vi "GetPressureAtMouse XYGraph.vi"(2 "Coords":T1, 3 "GraphRefnum":refnum<vi>) -> (0 "Numeric":dbl, 1 "String":string)   [LabVIEW 2013, in "main.lvlib"]
uses:
  main.lvlib
  <vilib>/Utility/miscctls.llb/LVPoint32TypeDef.ctl
  Controls/Enum Globals.ctl
  Controls/Enum Variables.ctl
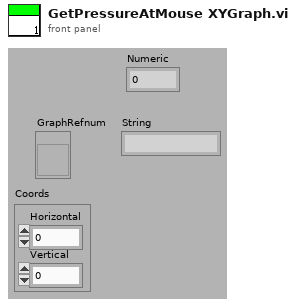
[diagram p1: front panel]
types:
  T1 = typedef "LVPoint32TypeDef.ctl" = cluster{"Horizontal":i32, "Vertical":i32}
  T2 = typedef "main.lvlib/Enum Variables.ctl" = enum16{"SetAcqFilter", "GetAcqFilter", "Set Filter", "Get Filter", "Set Height", "Get Height", "Set Blue Pressure", "Get Blue Pressure", "Set Red Pressure", "Get Red Pressure", "Init", "Reset Pressure", "Set Red Cursors", "Get Red Cursors", "Set Blue Cursors", "Get Blue Cursors", "Set Language", "Get Language", "Set Active Graphs", "Get ActiveGraphs", "Set Method", "Get Method", "Set Encryption", "Get Encryption", "Set ExcelVersion", "Get ExcelVersion", "Set DICOM Avail", "Get DICOM Avail", "Set DICOM Encode", "Get DICOM Encode", "Set JournalExport", "Get JournalExport", "Set Sequence", "Get Sequence", "Set DAQ Connected", "Get DAQ Connected", "Set Current Graph", "Get Current Graph", "Set General Settings", "Get Hyphenation", "Set Arm Calc Method", "Get Arm Calc Method", "Set Dicom Tags", "Get Dicom Tags", "Set BT Serial", "Get BT Serial", "Set BT Accepted Serials", "Get BT Accepted Serials", "Get BT License", "Set BT License"}
  T3 = typedef "main.lvlib/Enum Globals.ctl" = enum16{"Init", "Set DataPath", "Set Freq", "Get"}
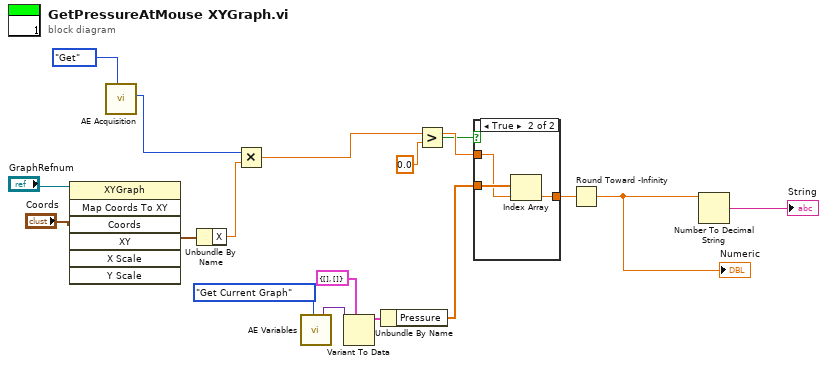
[diagram p0: block diagram]
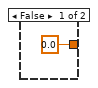
[diagram p2: hidden frame]
diagram:
  n1 = invoke class="XYGraph" method="Map Coords To XY"(reference="GraphRefnum", "Coords"="Coords") -> ("XY"=w14:cluster{"X":dbl, "Y":dbl})  [unwired: 5 in, 6 out]
  n2 = call "AE Acquisition.vi"("Action"=Enum_Globals."Get") -> ("Freq Out"=w7:i32)  [unwired: 7 in, 3 out]
  n3 = Unbundle By Name(w14) -> ("X"=w15:dbl)
  n4 = Multiply(x=w7, y=w15) -> (x*y=w12:dbl)
  n5 = call "AE Variables.vi"("Action"=Enum_Variables."Get Current Graph") -> ("Variant"=w3:variant)  [unwired: 11 in, 7 out]
  n6 = Variant To Data(type=cluster{"Pressure":dbl[], "Graph":dbl[]} {"Pressure"=[], "Graph"=[]}, Variant=w3) -> (data=w5:cluster{"Pressure":dbl[], "Graph":dbl[]})  [unwired: 1 in, 1 out]
  n7 = Unbundle By Name(w5) -> ("Pressure"=w1:dbl[])
  n8 = Greater?(x=w12, y=0.0) -> (0:w10:bool)
  n9 = case shown="True" w10 {
    tunnel: w1 -> [_ w21]
    tunnel: w12 -> [_ w20]
    tunnel: [0.0 w19] -> w13
    frame False {
    }
    frame True {
      n10 = Index Array(array=w21, index=w20) -> (element=w19:dbl)
    }
  }
  n11 = Round Toward -Infinity(1:w13) -> (0:w6:dbl)
  "Numeric" <- w6
  n12 = Number To Decimal String(number=w6) -> (decimal integer string=→"String":string)  [unwired: 1 in]
